vi "PID Table (Chien-Hrones-Reswick).vi"(5 "Tuning specifications":u16(ring) items=["Regulator - 0 %", "Regulator -  20%", "Servo - 0%", "Servo - 20%"], 7 "Type of Controller":u16(ring) items=["P", "PI", "PID"], 9 "Dead Time (L)":dbl, 10 "Time Constant (T)":dbl, 11 "Plant Gain (K)":dbl) -> (1 "Derivative Time (Td)":dbl, 2 "Integral Time (Ti)":dbl, 3 "Proportional Gain (Kp)":dbl)   [LabVIEW 2017, in "NI_PID_autopid.lvlib"]
uses:
  <vilib>/addons/control/pid/NI_PID_autopid.lvlib
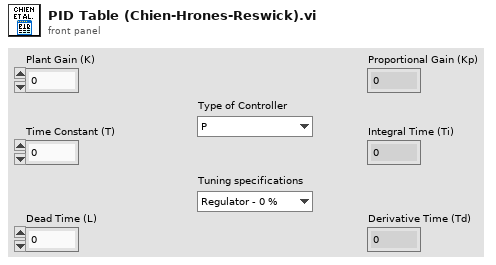
[diagram p1: front panel]
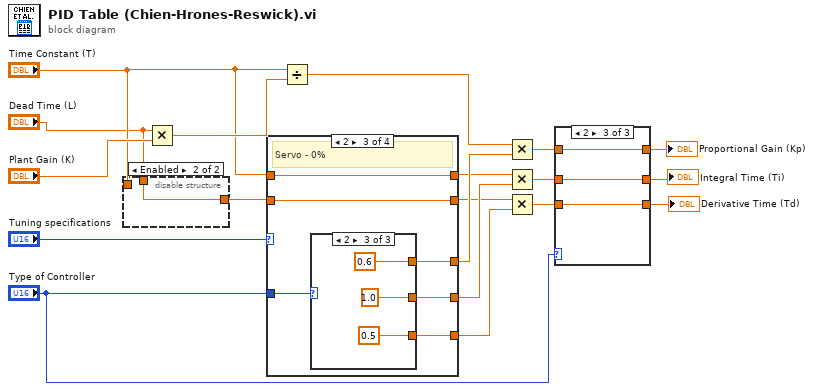
[diagram p0: block diagram]
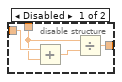
[diagram p2: hidden frame]
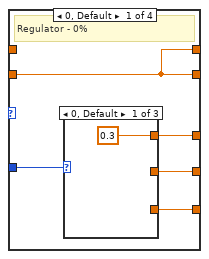
[diagram p3: hidden frame]
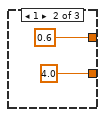
[diagram p4: hidden frame]
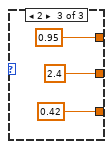
[diagram p5: hidden frame]
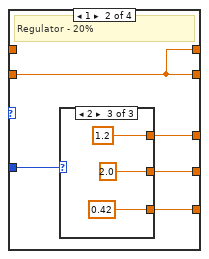
[diagram p6: hidden frame]
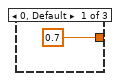
[diagram p7: hidden frame]
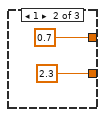
[diagram p8: hidden frame]
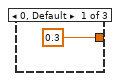
[diagram p9: hidden frame]
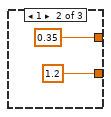
[diagram p10: hidden frame]
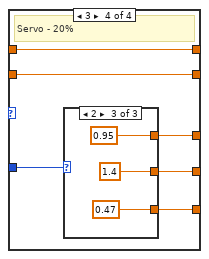
[diagram p11: hidden frame]
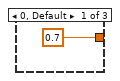
[diagram p12: hidden frame]
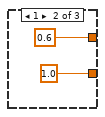
[diagram p13: hidden frame]
diagram:
  n1 = disable-structure shown="Enabled" {
    disable-tunnel: [w22 w24] -> w13
    disable-tunnel: "Time Constant (T)" -> [w21 _]
    disable-tunnel: "Dead Time (L)" -> [w20 w24]
    frame Disabled {
      n2 = Add(x=w21, y=w20) -> (x+y=w23:dbl)
      n3 = Divide(x=w20, y=w23) -> (x/y=w22:dbl)
    }
    frame Enabled {
    }
  }
  n4 = Multiply(x="Dead Time (L)", y="Plant Gain (K)") -> (x*y=w18:dbl)
  n5 = case shown="2" "Tuning specifications" {
    tunnel: "Type of Controller" -> [w29 w39 w52 w64]
    tunnel: [w28 w38 w51 w63] -> w16
    tunnel: w13 -> [w25 w40 w47 w59]
    tunnel: [w27 w37 w49 w61] -> w12
    tunnel: [w26 w36 w48 w60] -> w9
    tunnel: "Time Constant (T)" -> [_ _ w50 w62]
    tunnel: [w25 w40 w50 w62] -> w3
    tunnel: [w25 w40 w47 w59] -> w2
    frame 0, Default {
      # "Regulator - 0%"
      n6 = case shown="0, Default" w29 {
        tunnel: [0.3 ("Kp 6") 0.6 ("Kp 6") 0.95 ("Kp 6")] -> w28
        tunnel: [_ 4.0 ("Kp 6") 2.4 ("Kp 6")] -> w27
        tunnel: [_ _ 0.42 ("Kp 6")] -> w26
        frame 0, Default {
        }
        frame 1 {
        }
        frame 2 {
        }
      }
    }
    frame 1 {
      # "Regulator - 20%"
      n7 = case shown="2" w39 {
        tunnel: [0.7 ("Kp 6") 0.7 ("Kp 6") 1.2 ("Kp 6")] -> w38
        tunnel: [_ 2.3 ("Kp 6") 2.0 ("Kp 6")] -> w37
        tunnel: [_ _ 0.42 ("Kp 6")] -> w36
        frame 0, Default {
        }
        frame 1 {
        }
        frame 2 {
        }
      }
    }
    frame 2 {
      # "Servo - 0%"
      n8 = case shown="2" w52 {
        tunnel: [0.3 ("Kp 6") 0.35 ("Kp 6") 0.6 ("Kp 6")] -> w51
        tunnel: [_ 1.2 ("Kp 6") 1.0 ("Kp 6")] -> w49
        tunnel: [_ _ 0.5 ("Kp 6")] -> w48
        frame 0, Default {
        }
        frame 1 {
        }
        frame 2 {
        }
      }
    }
    frame 3 {
      # "Servo - 20%"
      n9 = case shown="2" w64 {
        tunnel: [0.7 ("Kp 6") 0.6 ("Kp 6") 0.95 ("Kp 6")] -> w63
        tunnel: [_ 1.0 ("Kp 6") 1.4 ("Kp 6")] -> w61
        tunnel: [_ _ 0.47 ("Kp 6")] -> w60
        frame 0, Default {
        }
        frame 1 {
        }
        frame 2 {
        }
      }
    }
  }
  n10 = Divide(x="Time Constant (T)", y=w18) -> (x/y=w15:dbl)
  n11 = Multiply(x=w15, y=w16) -> (x*y=w5:dbl)
  n12 = Multiply(x=w3, y=w12) -> (x*y=w10:dbl)
  n13 = Multiply(x=w2, y=w9) -> (x*y=w8:dbl)
  n14 = case shown="2" "Type of Controller" {
    tunnel: w5 -> [w71 w73 w76]
    tunnel: [w71 w73 w76] -> w14
    tunnel: [_ w72 w74] -> w11
    tunnel: w10 -> [_ w72 w74]
    tunnel: w8 -> [_ _ w75]
    tunnel: [_ _ w75] -> w7
    frame 0, Default {
    }
    frame 1 {
    }
    frame 2 {
    }
  }
  "Proportional Gain (Kp)" <- w14
  "Integral Time (Ti)" <- w11
  "Derivative Time (Td)" <- w7
